vi "Set Meta Data.vi"(7 "Unique ID":string, 8 "error in (no error)":errorcluster, 10 "Meta Data":string, 11 "Test Executive in":refnum<class "Test Executive.lvclass">) -> (0 "error out":errorcluster, 3 "Test Executive out":refnum<class "Test Executive.lvclass">)   [LabVIEW 2017, in "Test Executive.lvlib" / "Test Executive.lvclass"]
uses:
  <vilib>/gpm_packages/@cs/test-executive/Source/Test Executive/TestExecutive/Test Executive.lvclass
  <vilib>/gpm_packages/@cs/test-executive/Source/Test Executive/TestExecutive/Test Executive.lvclass/Test Executive.ctl
  <vilib>/gpm_packages/@cs/linked-list/Source/Linked List/Linked List Ref/Linked List Ref.lvclass
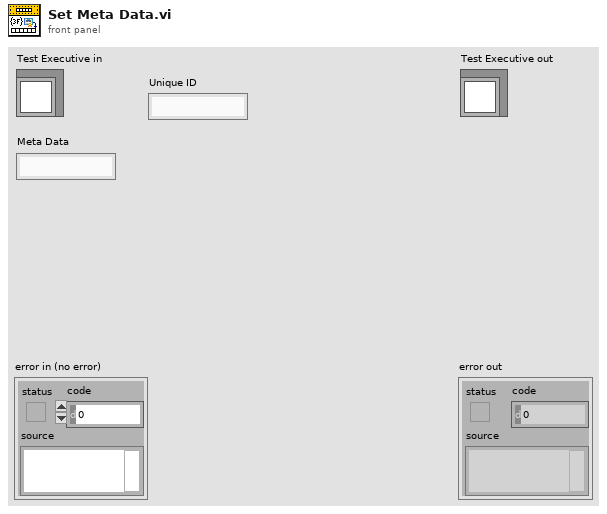
[diagram p1: front panel]
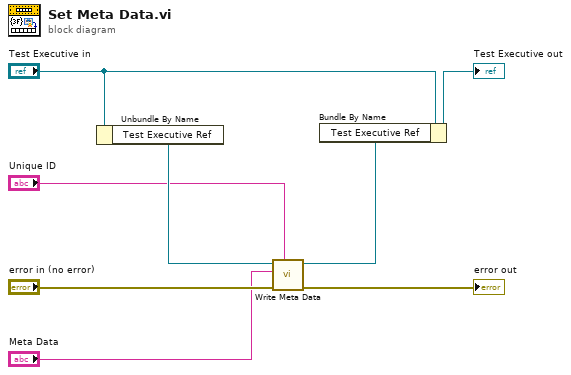
[diagram p0: block diagram]
diagram:
  n1 = Unbundle By Name("Test Executive in") -> ("Test Executive Ref"=w7:refnum<data-value>)
  n2 = call <vilib>:"Write Meta Data.vi"("Linked List ID"="Unique ID", "error in (no error)"="error in (no error)", "Meta Data"="Meta Data", "Linked List Ref"=w7) -> ("error out"=→"error out":errorcluster, "Linked List Ref out"=w3:refnum<data-value>)  [unwired: 5 in, 1 out]
  n3 = Bundle By Name(cluster="Test Executive in", "Test Executive Ref"=w3) -> (→"Test Executive out":refnum<class "Test Executive.lvclass">)
